vi "Simple Add.vi"() -> ()   [LabVIEW 2015]
panel:
  out "x+y":dbl
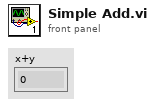
[diagram p1: front panel]
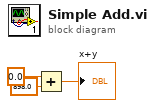
[diagram p0: block diagram]
diagram:
  n1 = Add(x=0.0, y=898.0) -> (x+y=→"x+y":dbl)
